vi "Read Panel1.vi"(8 "error in (no error)":errorcluster, 11 "Bouncer in":refnum<class "Bouncer.lvclass">) -> (0 "error out":errorcluster, 2 "RT_Game.lvlib:BouncePanel.lvclass":refnum<class "BouncePanel.lvclass">, 3 "Bouncer out":refnum<class "Bouncer.lvclass">)   [LabVIEW 2019, in "RT_Game.lvlib" / "Bouncer.lvclass"]
uses:
  Bouncer.lvclass
  BouncePanel/BouncePanel.lvclass
  Bouncer.lvclass/Bouncer.ctl
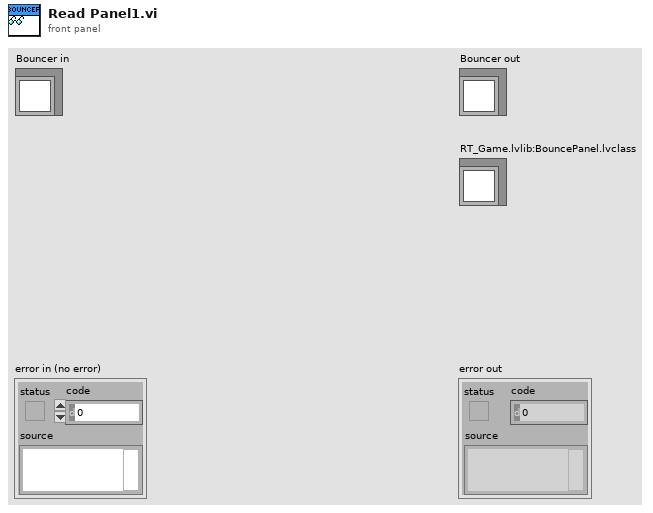
[diagram p1: front panel]
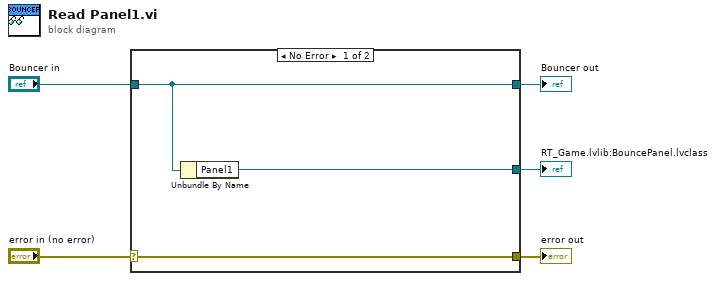
[diagram p0: block diagram]
diagram:
  n1 = case shown="No Error" "error in (no error)" {
    selector: "error in (no error)" -> [w8 w9]
    tunnel: [w8 w9] -> w4
    tunnel: [w7 w10] -> w2
    tunnel: "Bouncer in" -> [w7 w10]
    tunnel: [w6 _] -> w1
    frame No Error {
      n2 = Unbundle By Name(w7) -> ("Panel1"=w6:refnum<class "BouncePanel.lvclass">)
    }
    frame Error {
    }
  }
  "error out" <- w4
  "Bouncer out" <- w2
  "RT_Game.lvlib:BouncePanel.lvclass" <- w1
